vi "Trigger VI.vi"() -> ()   [LabVIEW 2021]
uses:
  <instrlib>/Tektronix TDS 200 1000 2000 Series/Public/Configure/Configure Trigger (Edge).vi
  <instrlib>/Tektronix TDS 200 1000 2000 Series/Tektronix TDS 200 1000 2000 Series.lvlib
panel:
  in  "OK Button":bool
  in  "Trigger Coupling (0: AC)":i32(ring) items=["AC", "DC", "HF Reject", "LF Reject", "Noise Reject"]
  in  "Trigger Slope (0: Rising)":i32(ring) items=["Rising", "Falling"]
  in  "Holdoff (0.00)":dbl format="%_3g"
  in  "Trigger Mode (0: Auto)":i32(ring) items=["Auto", "Normal"]
  in  "Trigger Level (0.0 V)":dbl
  in  "Trigger Source (0: Channel 1)":i32(ring) items=["Channel 1", "Channel 2", "Channel 3", "Channel 4", "External Input", "Attenuated External Input"]
  in  "CH2":bool
  in  "CH1":bool
  out "XY Graph":cluster{"Y":dbl[], "Y":dbl[]}(graph)
  out "Waveform Graph":waveform(dbl)[](graph)
  in  "VISA resource name":refnum<visa-resource-name>
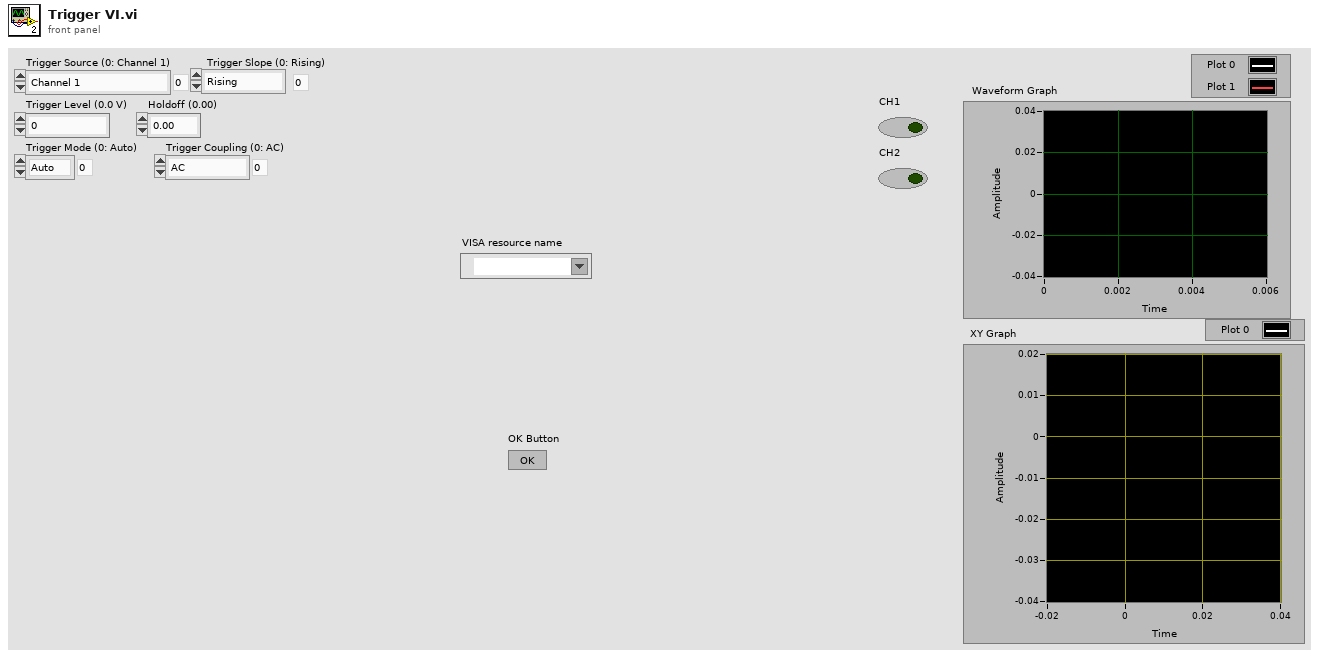
[diagram p1: front panel]
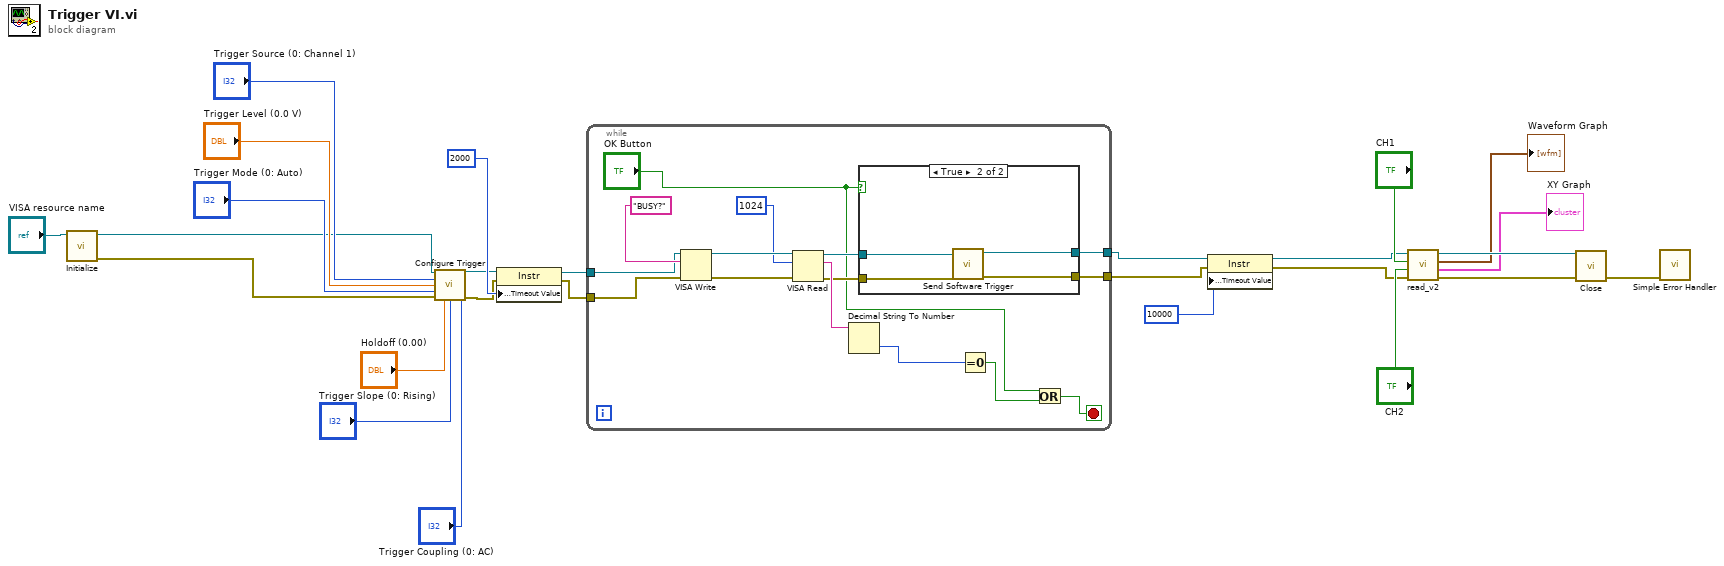
[diagram p0: block diagram]
diagram:
  n1 = call <instrlib>:"Initialize.vi"("VISA resource name"="VISA resource name") -> ("error out"=w12:errorcluster, "VISA resource name out"=w13:refnum<visa-resource-name>)  [unwired: 9 in]
  n2 = call-poly <instrlib>:"Configure Trigger.vi"("VISA resource name"=w13, "Trigger Source (0: Channel 1)"="Trigger Source (0: Channel 1)", "Trigger Level (0.0 V)"="Trigger Level (0.0 V)", "Trigger Mode (0: Auto)"="Trigger Mode (0: Auto)", "error in (no error)"=w12, "Holdoff (0.00)"="Holdoff (0.00)", "Trigger Slope (0: Rising)"="Trigger Slope (0: Rising)", "Trigger Coupling (0: AC)"="Trigger Coupling (0: AC)") -> ("VISA resource name out"=w8:refnum<visa-resource-name>, "error out"=w7:errorcluster)  [unwired: 6 in]
  n3 = property class="Instr"(reference=w8, error in=w7, "General Settings:Timeout Value"=u32 2000) -> (reference out=w10:refnum<visa-resource-name>, error out=w9:errorcluster)
  n4 = while {
    tunnel: [w31] -> w5
    tunnel: [w30] -> w4
    tunnel: w10 -> [w29]
    tunnel: w9 -> [w28]
    stop <- w35 stop-if-true
    n5 = VISA Write(VISA resource name=w29, write buffer="BUSY?", error in (no error)=w28) -> (VISA resource name out=w40:refnum<visa-resource-name>, error out=w39:errorcluster)  [unwired: 1 out]
    n6 = VISA Read(VISA resource name=w40, byte count=u32 1024, error in (no error)=w39) -> (VISA resource name out=w33:refnum<visa-resource-name>, read buffer=w36:string, error out=w32:errorcluster)  [unwired: 1 out]
    n7 = Decimal String To Number(string=w36) -> (number=w37:i32)  [unwired: 2 in, 1 out]
    n8 = case shown="True" "OK Button" {
      tunnel: w33 -> [w43 w47]
      tunnel: w32 -> [w42 w46]
      tunnel: [w43 w45] -> w31
      tunnel: [w42 w44] -> w30
      frame False {
      }
      frame True {
        n9 = call <instrlib>:"Send Software Trigger.vi"("error in (no error)"=w46, "VISA resource name"=w47) -> ("error out"=w44:errorcluster, "VISA resource name out"=w45:refnum<visa-resource-name>)  [unwired: 8 in]
      }
    }
    n10 = Equal To 0?(x=w37) -> (x = 0?=w34:bool)
    n11 = Or(x="OK Button", y=w34) -> (x .or. y?=w35:bool)
  }
  n12 = property class="Instr"(reference=w5, error in=w4, "General Settings:Timeout Value"=u32 10000) -> (reference out=w3:refnum<visa-resource-name>, error out=w2:errorcluster)
  n13 = call "read_v2.vi"("error in (no error)"=w2, "Boolean 2"="CH2", "Boolean"="CH1", "VISA resource name"=w3) -> ("error out"=w25:errorcluster, "XY Graph"=→"XY Graph":cluster{"Y":dbl[], "Y":dbl[]}, "Waveform Graph"=→"Waveform Graph":waveform(dbl)[], "VISA resource name out"=w26:refnum<visa-resource-name>)  [unwired: 4 in]
  n14 = call <instrlib>:"Close.vi"("error in (no error)"=w25, "VISA resource name"=w26) -> ("error out"=w1:errorcluster)  [unwired: 9 in]
  n15 = call <vilib>:"Simple Error Handler.vi"("error in (no error)"=w1) -> ()  [unwired: 4 in, 5 out]
